vi "KepcoDCPwr Configure Voltage Limit.vi"(0 "VISA Session":refnum<visa-resource-name>, 5 "Model In":string, 7 "channel name (\"\")":string="\"\"", 11 "error in (no error)":errorcluster {"code" format="%.0x"}, 12 "limit (0.0)":dbl format="%^.2e") -> (4 "VISA Session Out":refnum<visa-resource-name>, 6 "Model Out":string, 8 "channel name out (\"\")":string="\"\"" caption="channel name Out (\"\")", 15 "error out":errorcluster {"code" format="%.0x"})   [LabVIEW 2013]
doc: "This VI configures the output voltage limit.\n\nThis limit prevents VOLT settings abovethe limit value. \nNOTE, Does not support for Bipolar limits of BOP 1000 Watt unit and BOP A unit.\nUse Configure Both voltage Limits for bipolar limit settings."
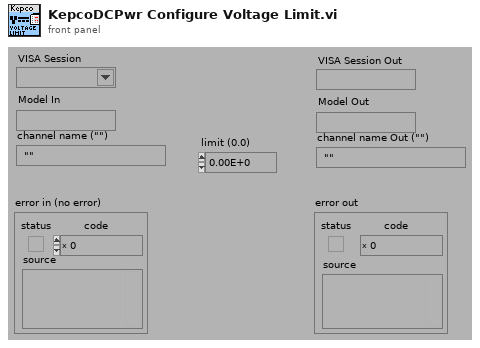
[diagram p1: front panel]
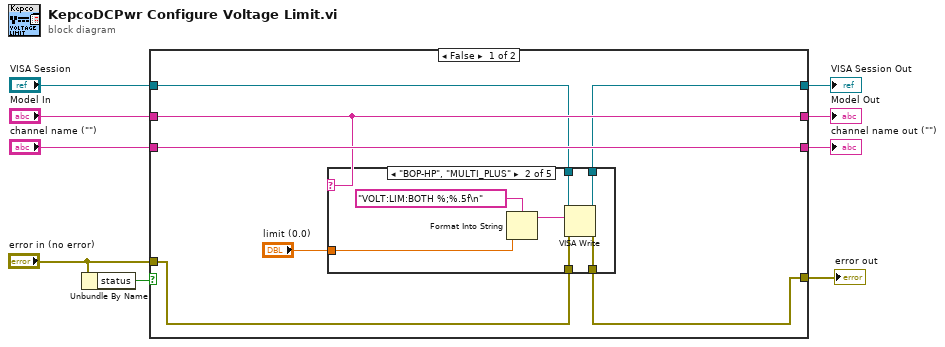
[diagram p0: block diagram]
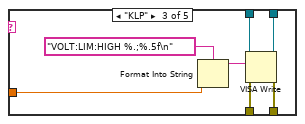
[diagram p3: hidden frame]
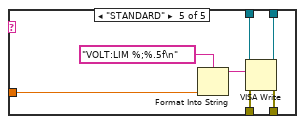
[diagram p5: hidden frame]
diagram:
  n1 = Unbundle By Name("error in (no error)") -> ("status"=w6:bool)
  n2 = case shown="False" w6 {
    tunnel: [w12 w44] -> w9
    tunnel: [w13 w45] -> w7
    tunnel: "VISA Session" -> [w14 w45]
    tunnel: "error in (no error)" -> [w11 w44]
    tunnel: "Model In" -> [w15 w43]
    tunnel: [w15 w43] -> w1
    tunnel: "channel name (\"\")" -> [w16 w42]
    tunnel: [w16 w42] -> w2
    frame False {
      n3 = case shown="\"BOP-HP\", \"MULTI_PLUS\"" w15 {
        tunnel: w11 -> [w18 w25 w31 w33 w36]
        tunnel: [w18 w24 w30 w33 w35] -> w12
        tunnel: w14 -> [w17 w23 w32 w34 w38]
        tunnel: [w17 w22 w29 w34 w37] -> w13
        tunnel: "limit (0.0)" -> [_ w20 w26 _ w39]
        frame "", Default {
        }
        frame "BOP-HP", "MULTI_PLUS" {
          n4 = Format Into String(format string="VOLT:LIM:BOTH %;%.5f\n", w20) -> (resulting string=w21:string)  [unwired: 2 in, 1 out]
          n5 = VISA Write(VISA resource name=w23, write buffer=w21, error in (no error)=w25) -> (VISA resource name out=w22:refnum<visa-resource-name>, error out=w24:errorcluster)  [unwired: 1 out]
        }
        frame "KLP" {
          n6 = Format Into String(format string="VOLT:LIM:HIGH %.;%.5f\n", w26) -> (resulting string=w27:string)  [unwired: 2 in, 1 out]
          n7 = VISA Write(VISA resource name=w32, write buffer=w27, error in (no error)=w31) -> (VISA resource name out=w29:refnum<visa-resource-name>, error out=w30:errorcluster)  [unwired: 1 out]
        }
        frame "BOP-LP", "MULTI" {
        }
        frame "STANDARD" {
          n8 = Format Into String(format string="VOLT:LIM %;%.5f\n", w39) -> (resulting string=w40:string)  [unwired: 2 in, 1 out]
          n9 = VISA Write(VISA resource name=w38, write buffer=w40, error in (no error)=w36) -> (VISA resource name out=w37:refnum<visa-resource-name>, error out=w35:errorcluster)  [unwired: 1 out]
        }
      }
    }
    frame True {
    }
  }
  "error out" <- w9
  "VISA Session Out" <- w7
  "channel name out (\"\")" <- w2
  "Model Out" <- w1
